vi "WPI_CameraConvert Version String to Header String.vi"(7 "String":string) -> (8 "string":string)   [LabVIEW 2017]
doc: "Converts an input string of the form \"a.b.c.d\" into a string of the form \"ABCD\", where a,b,c,d are integers in the range 0-255 and A, B, C, D are the characters whose ascii values are a,b,c,d respectively. \n\nUse this VI to create the version string to send before you transfer image data to the PC. \n\nThis software is licensed. Open the labview\\readme\\WPI Robotics Library Open Source License.txt file for more information."
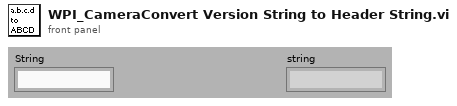
[diagram p1: front panel]
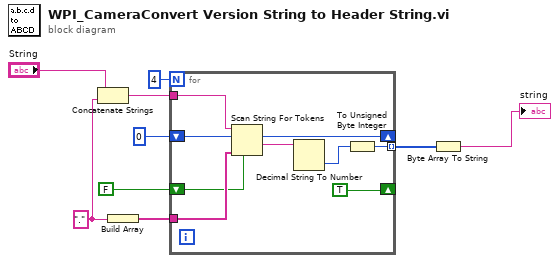
[diagram p0: block diagram]
diagram:
  w6 = "."
  n1 = Concatenate Strings("String", w6) -> (w7:string)
  n2 = Build Array(w6) -> (w2:string[])
  n3 = for {
    N: 4 -> [_]
    shift-right: [TRUE] -> _
    shift-left: FALSE -> [w15]
    shift-right: [w10] -> _
    shift-left: 0 -> [w11]
    tunnel: w2 -> [w16]
    tunnel: [w13] -> w3 mode=indexing
    tunnel: w7 -> [w12]
    n4 = Scan String For Tokens(4:w15, 6:w16, 8:w11, 9:w12) -> (1:w17:string, 2:w10:i32)  [unwired: 4 out]
    n5 = Decimal String To Number(string=w17) -> (number=w14:i32)  [unwired: 3 out]
    n6 = To Unsigned Byte Integer(number=w14) -> (unsigned 8bit integer=w13:u8)
  }
  n7 = Byte Array To String(unsigned byte array=w3) -> (string=→"string":string)
